vi "Periodic Tasks.vi"(8 "error in":errorcluster) -> ()   [LabVIEW 2018]
doc: "This VI runs in parallel to other tasks. It can contain as many user-defined periodic loops as you need. These can carry out PID or other sorts of timed response."
uses:
  <vilib>/Rock Robotics/WPI/ThirdParty/Sensors/navX/_TypeDefs/FRIC_navX_DeviceNumbersTypeDef.ctl
  <vilib>/Rock Robotics/WPI/DriverStation/WPI_DriverStationDerivedRobotMode.ctl
  <vilib>/Rock Robotics/WPI/DriverStation/WPI_DriverStationRobotMode2.ctl
  <vilib>/Rock Robotics/WPI/ThirdParty/Sensors/navX/_Processing Loop/FRIC_navX_Internal_SPI_ProcessingLoop.vi
  Robot Global Data.vi
  SubSystems/Robot Information/Robot Information Global.vi
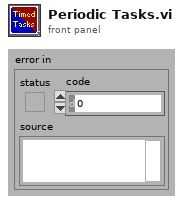
[diagram p1: front panel]
types:
  T1 = typedef "FRIC_navX_DeviceNumbersTypeDef.ctl" = enum16{"Dev0", "Dev1", "Dev2", "Dev3"}
  T2 = typedef "WPI_DriverStationRobotMode2.ctl" = enum16{"Autonomous Disabled", "Autonomous Enabled", "Teleop Disabled", "Teleop Enabled", "Disconnected", "Finish", "Test Disabled", "Test Enabled", "Emergency Stopped"}
  T3 = typedef "WPI_DriverStationDerivedRobotMode.ctl" = enum16{"Init", "Execute", "Stop"}
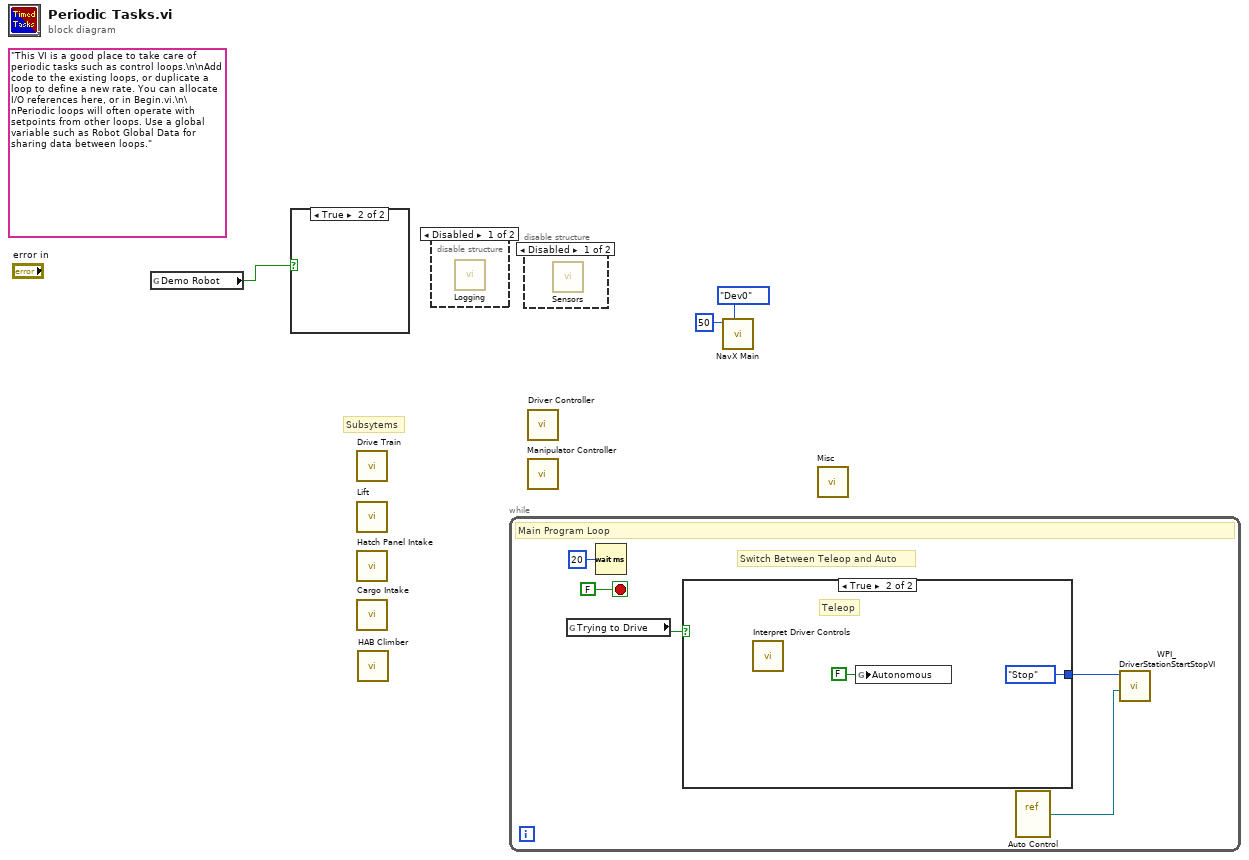
[diagram p0: block diagram]
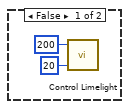
[diagram p2: hidden frame]
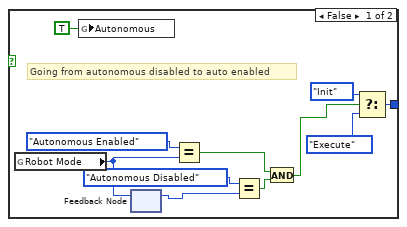
[diagram p3: hidden frame]
diagram:
  (unwired) "This VI is a good place to take care of periodic tasks such as control loops.\n\nAdd code to the existing loops, or duplicate a loop to define a new rate. You can allocate I/O references here, or in Begin.vi.\n\nPeriodic loops will often operate with setpoints from other loops. Use a global variable such as Robot Global Data for sharing data between loops."
  # "Subsytems"
  n1 = global read "Robot Information Global.vi" "Demo Robot"() -> (w1:bool)
  n2 = case shown="True" w1 {
    frame False {
      n3 = call "Control Limelight.vi"("Read Data Loop Time (ms) (min 10)"=u32 20, "Write Data Loop Time (ms)"=u32 200) -> ()  [unwired: 1 in]
    }
    frame True {
    }
  }
  n4 = call "Drive Train.vi"() -> ()  [unwired: 12 in]
  n5 = call "Lift.vi"() -> ()  [unwired: 1 in]
  n6 = call "Hatch Panel Intake.vi"() -> ()  [unwired: 10 in]
  n7 = call "Cargo Intake.vi"() -> ()  [unwired: 12 in]
  n8 = call "HAB Climber.vi"() -> ()  [unwired: 12 in]
  n9 = disable-structure shown="Disabled" {
    frame Disabled {
      n10 = call "Logging.vi"() -> ()  [unwired: 12 in]
    }
    frame Enabled {
    }
  }
  n11 = while {
    stop <- FALSE stop-if-true
    # "Switch Between Teleop and Auto"
    # "Main Program Loop"
    n12 = global read "Robot Global Data.vi" "Trying to Drive"() -> (w8:bool)
    n13 = Wait (ms)(milliseconds to wait=u32 20) -> ()  [unwired: 1 out]
    n14 = case shown="True" w8 {
      tunnel: [w20 WPI_DriverStationDerivedRobotMode."Stop" ("f")] -> w7
      frame False {
        # "Going from autonomous disabled to auto enabled"
        n15 = global read "Robot Global Data.vi" "Robot Mode"() -> (w17:T2)
        n16 = global write "Robot Global Data.vi" "Autonomous"(TRUE ("Autonomous")) -> ()
        n17 = feedback #1() -> (w14:T2)  [unwired: 1 in]
        n18 = feedback-in #1(w17) -> ()
        n19 = Equal?(x=WPI_DriverStationRobotMode2."Autonomous Enabled" ("y"), y=w17) -> (x = y?=w12:bool)
        n20 = Equal?(x=WPI_DriverStationRobotMode2."Autonomous Disabled" ("y"), y=w14) -> (x = y?=w13:bool)
        n21 = And(x=w12, y=w13) -> (x .and. y?=w11:bool)
        n22 = Select(t=WPI_DriverStationDerivedRobotMode."Init" ("Call Context"), s=w11, f=WPI_DriverStationDerivedRobotMode."Execute") -> (s? t:f=w20:T3)
      }
      frame True {
        # "Teleop"
        n23 = call "Interpret Driver Controls.vi"() -> ()  [unwired: 12 in]
        n24 = global write "Robot Global Data.vi" "Autonomous"(FALSE ("Autonomous")) -> ()
      }
    }
    n25 = vi-ref "Auto Control.vi"() -> (w6:refnum<vi>)
    n26 = call <vilib>:"WPI_DriverStationStartStopVI.vi"("VI in"=w6, "Call Context"=w7) -> ()  [unwired: 10 in]
  }
  n27 = disable-structure shown="Disabled" {
    frame Disabled {
      n28 = call "Sensors.vi"() -> ()  [unwired: 12 in]
    }
    frame Enabled {
    }
  }
  n29 = call "Driver Controller.vi"() -> ()  [unwired: 12 in]
  n30 = call "Manipulator Controller.vi"() -> ()  [unwired: 12 in]
  n31 = call-poly <vilib>:"NavX Main.vi"("Device Number"=FRIC_navX_DeviceNumbersTypeDef."Dev0", "Rate (4Hz-200Hz)"=u8 50) -> ()  [unwired: 10 in]
  n32 = call "Misc.vi"() -> ()  [unwired: 12 in]
